vi "Relatorio_Variaveis.vi"() -> ()   [LabVIEW 2019]
panel:
  in  "ListRelatorios":string[](array[string])
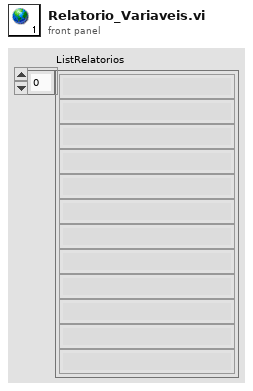
[diagram p1: front panel]
diagram:
